vi "Scoring Manager Async.vi"(10 "Pool Size":i32=2, 11 "SOL-Server in":refnum<class "SOL-Server.lvclass">) -> ()   [LabVIEW 2020, in "Summer of LabVIEW.lvlib" / "SOL-Server.lvclass"]
uses:
  SOL-Server.lvclass
  SOL-Server.lvclass/SOL-Server.ctl
  Scorer/Scorer.lvclass
panel:
  out "Working":bool[](array[boolean])
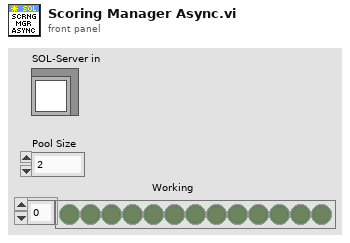
[diagram p1: front panel]
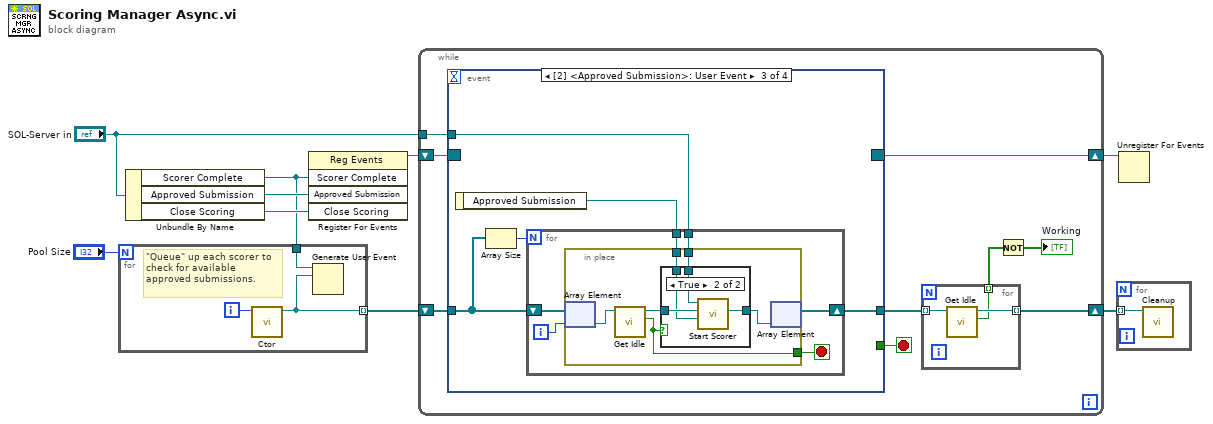
[diagram p0: block diagram]
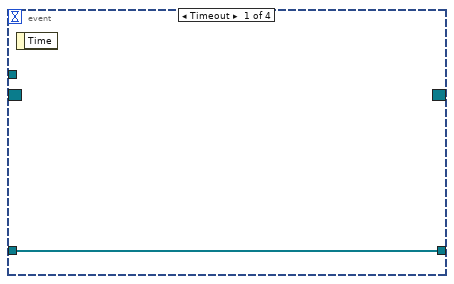
[diagram p2: hidden frame]
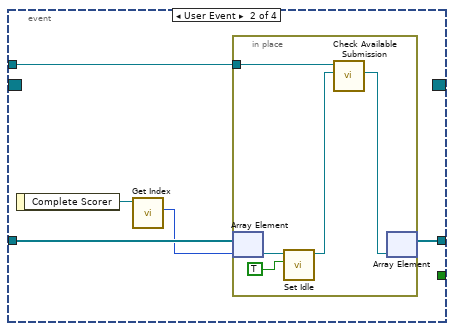
[diagram p3: hidden frame]
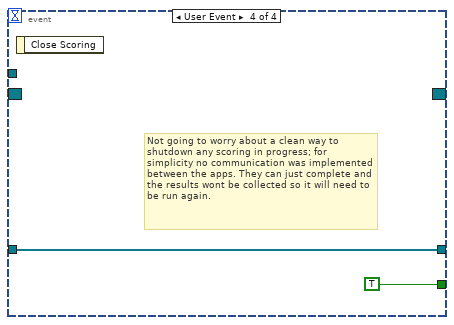
[diagram p5: hidden frame]
diagram:
  n1 = Unbundle By Name("SOL-Server in") -> ("Scorer Complete"=w2:refnum<user-event>, "Approved Submission"=w8:refnum<user-event>, "Close Scoring"=w5:refnum<user-event>)
  n2 = for {
    N: "Pool Size" -> [_]
    tunnel: [w10] -> w6 mode=indexing
    tunnel: w2 -> [w11]
    i -> [w12]
    # "\"Queue\" up each scorer to check for available approved submissions."
    n3 = call "Ctor.vi"("Index"=w12) -> ("Scorer out"=w10:refnum<class "Scorer.lvclass">)  [unwired: 9 in, 1 out]
    n4 = Generate User Event(user event=w11, event data cluster=w10) -> ()  [unwired: 2 in, 2 out]
  }
  n5 = register-events(w2, w8, w5) -> (reference out=w7:refnum<event-registration>)  [unwired: 2 in, 1 out]
  n6 = while {
    shift-right: [w20] -> w3
    shift-left: w7 -> [w21]
    shift-right: [w15] -> w1
    shift-left: w6 -> [w19]
    tunnel: "SOL-Server in" -> [w18]
    stop <- w17 stop-if-true
    n7 = event shown="[2] <Approved Submission>: User Event" {
      selector: w21 -> [_ _ _ _]
      dyn-events: [_ _ _ _] -> w20
      timeout: _ -> [_ _ _ _]
      tunnel: w19 -> [w22 w26 w33 w55]
      tunnel: w18 -> [_ w24 w37 _]
      tunnel: [w22 w23 w35 w55] -> w16
      tunnel: [_ _ _ TRUE] -> w17
      event Timeout {
        n8 = event-data() -> ()  [unwired: 1 in, 1 out]
      }
      event User Event {
        n9 = event-data() -> ("Complete Scorer"=w27:refnum<class "Scorer.lvclass">)  [unwired: 1 in]
        n10 = call "Get Index.vi"("Scorer in"=w27) -> ("Index"=w25:i32)  [unwired: 8 in, 2 out]
        n11 = in-place {
          in-place-border: w24 -> [w32]
          n12 = in-place-array #1(w26, w25) -> (w31:refnum<class "Scorer.lvclass">)
          n13 = call "Set Idle.vi"("Idle"=TRUE, "Scorer in"=w31) -> ("Scorer out"=w29:refnum<class "Scorer.lvclass">)  [unwired: 8 in, 1 out]
          n14 = call "Check Available Submission.vi"("Scorer In"=w29, "SOL-Server in"=w32) -> ("Scorer"=w28:refnum<class "Scorer.lvclass">)  [unwired: 7 in, 2 out]
          n15 = in-place-array #1(w28) -> (w23:refnum<class "Scorer.lvclass">[])  [unwired: 1 out]
        }
      }
      event User Event {
        n16 = event-data() -> ("Approved Submission"=w36:refnum<class "Submission.lvclass">)  [unwired: 1 in]
        n17 = Array Size(array=w33) -> (size(s)=w34:i32)
        n18 = for {
          N: w34 -> [_]
          tunnel: w37 -> [w43]
          tunnel: w36 -> [w42]
          shift-right: [w38] -> w35
          shift-left: w33 -> [w41]
          i -> [w40]
          stop <- w39 stop-if-true
          n19 = in-place {
            in-place-border: w43 -> [w48]
            in-place-border: w42 -> [w47]
            in-place-border: [w44] -> w39
            n20 = in-place-array #2(w41, w40) -> (w46:refnum<class "Scorer.lvclass">)
            n21 = call "Get Idle.vi"("Scorer in"=w46) -> ("Idle"=w44:bool, "Scorer out"=w49:refnum<class "Scorer.lvclass">)  [unwired: 8 in, 1 out]
            n22 = case shown="True" w44 {
              tunnel: w49 -> [w50 w53]
              tunnel: w48 -> [_ w54]
              tunnel: w47 -> [_ w51]
              tunnel: [w50 w52] -> w45
              frame False {
              }
              frame True {
                n23 = call "Start Scorer.vi"("Submission"=w51, "Scorer In"=w53, "SOL-Server in"=w54) -> ("Scorer"=w52:refnum<class "Scorer.lvclass">)  [unwired: 6 in, 2 out]
              }
            }
            n24 = in-place-array #2(w45) -> (w38:refnum<class "Scorer.lvclass">[])  [unwired: 1 out]
          }
        }
      }
      event User Event {
        # "Not going to worry about a clean way to shutdown any scoring in progress; for simplicity no communication was implemented between the apps. They can just complete and the results wont be collected so it will need to be run again."
        n25 = event-data() -> ()  [unwired: 1 in, 1 out]
      }
    }
    n26 = for {
      tunnel: w16 -> [w59] mode=indexing
      tunnel: [w58] -> w15 mode=indexing
      tunnel: [w57] -> w14 mode=indexing
      n27 = call "Get Idle.vi"("Scorer in"=w59) -> ("Idle"=w57:bool, "Scorer out"=w58:refnum<class "Scorer.lvclass">)  [unwired: 8 in, 1 out]
    }
    n28 = Not(x=w14) -> (.not. x?=→"Working":bool[])
  }
  n29 = for {
    tunnel: w1 -> [w60] mode=indexing
    n30 = call "Cleanup.vi"("Scorer in"=w60) -> ()  [unwired: 10 in, 1 out]
  }
  n31 = Unregister For Events(event registration refnum=w3) -> ()  [unwired: 1 in, 1 out]
